vi "e.gate Cleanup.vi"(8 "error in (no error)":errorcluster, 11 "e.gate Configuration":T1 {"dActTimeToSecondFactor" format="%#.10f"; "StartTimeToDayFactor" format="%#.10f"; "BufferFillRate" format="%#_10f"}) -> (0 "error out":errorcluster)   [LabVIEW 2016]
doc: "<B>AMC - Analytik & Messtechnik GmbH Chemnitz</B>\n\nLabVIEW Drivers for e.gate / e.pac series from Gantner Instruments\n\nThis VI closes the TCP/IP interface specified by <B>connection ID</B>. An incoming error is ignored but forwarded."
uses:
  e.gate Configuration.ctl
  e.gate Channel Data.ctl
  e.gate Data Type.ctl
  e.gate Protocol Type.ctl
  e.gate Module  Data.ctl
  e.gateHSP_DLLhandle.ctl
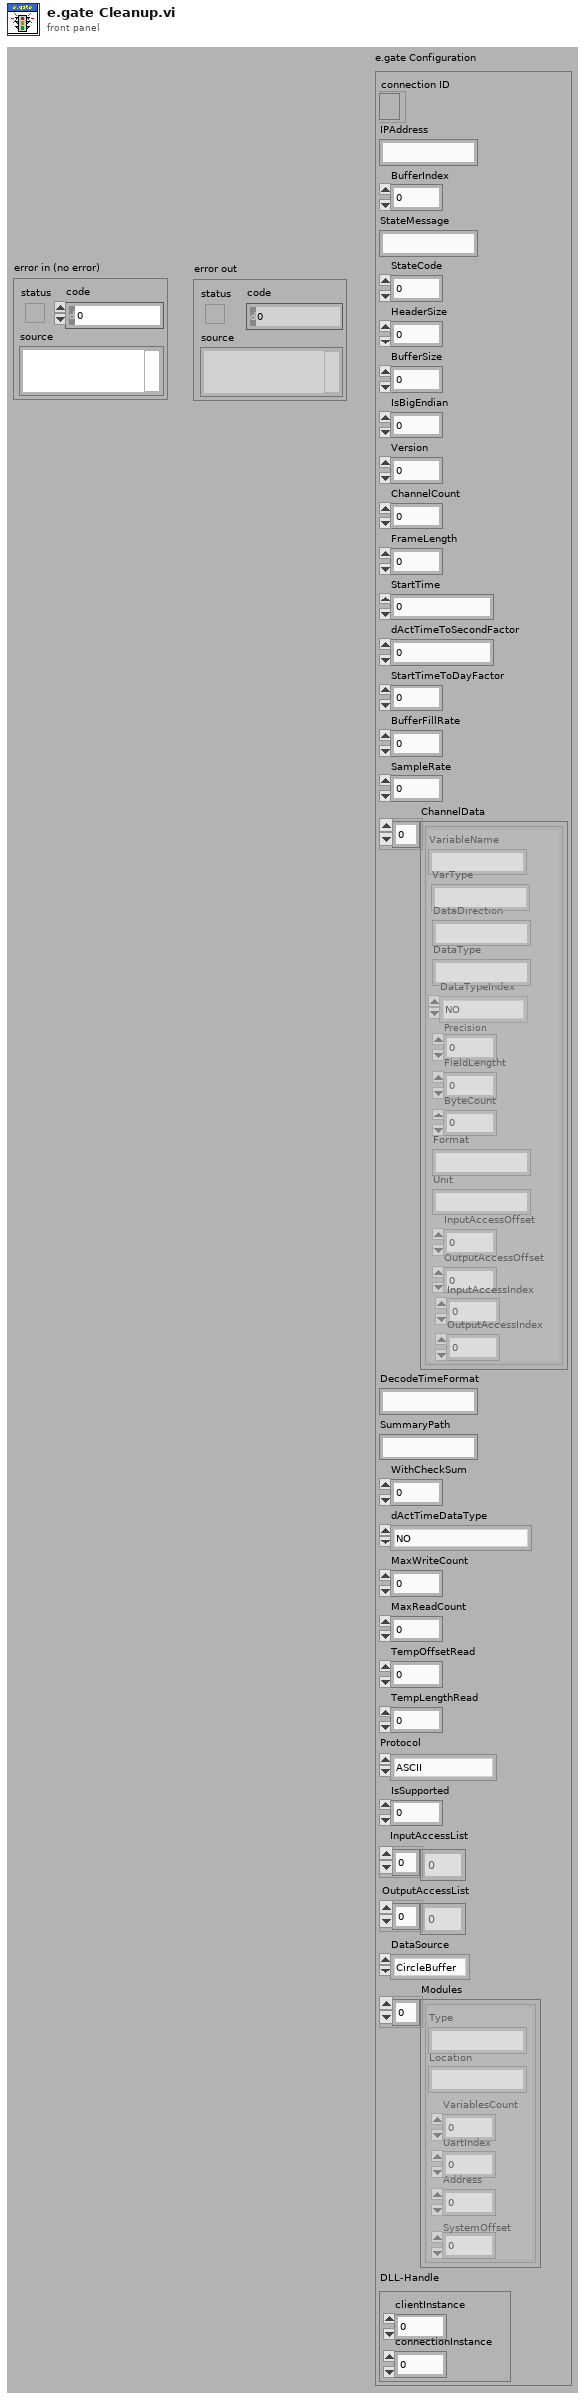
[diagram p1: front panel]
types:
  T1 = typedef "e.gate Configuration.ctl" = cluster{"connection ID":refnum<k5>, "IPAddress":string, "BufferIndex":i32, "StateMessage":string, "StateCode":i8, "HeaderSize":i32, "BufferSize":i32, "IsBigEndian":i32, "Version":i32, "ChannelCount":i32, "FrameLength":i32, "StartTime":dbl, "dActTimeToSecondFactor":dbl, "StartTimeToDayFactor":dbl, "BufferFillRate":dbl, "SampleRate":dbl, "ChannelData":T2[], "DecodeTimeFormat":string, "SummaryPath":string, "WithCheckSum":i32, "dActTimeDataType":T3, "MaxWriteCount":i32, "MaxReadCount":i32, "TempOffsetRead":i32, "TempLengthRead":i32, "Protocol":T4, "IsSupported":i32, "InputAccessList":i32[], "OutputAccessList":i32[], "DataSource":enum16{"CircleBuffer", "test.con Logger", "test.con Archive"}, "Modules":T5[], "DLL-Handle":T6}
  T2 = typedef "e.gate Channel Data.ctl" = cluster{"VariableName":string, "DataDirection":string, "DataType":string, "DataTypeIndex":T3, "Precision":i16, "FieldLengtht":i16, "ByteCount":i32, "Format":string, "Unit":string, "InputAccessOffset":i32, "OutputAccessOffset":i16, "InputAccessIndex":i16, "OutputAccessIndex":i16, "VarType":string}
  T3 = typedef "e.gate Data Type.ctl" = enum16{"NO", "BOOL", "SINT8", "USINT8", "SINT16", "USINT16", "SINT32", "USINT32", "FLOAT", "SET8", "SET16", "SET32", "DOUBLE", "SINT64", "USINT64", "SET64"}
  T4 = typedef "e.gate Protocol Type.ctl" = enum16{"ASCII", "HighspeedPort Online", "HighspeedPort Buffer", "eGateHighspeedPortDLL "}
  T5 = typedef "e.gate Module  Data.ctl" = cluster{"Type":string, "Location":string, "VariablesCount":i16, "UartIndex":i16, "Address":i16, "SystemOffset":i16}
  T6 = typedef "e.gateHSP_DLLhandle.ctl" = cluster{"clientInstance":i32, "connectionInstance":i32}
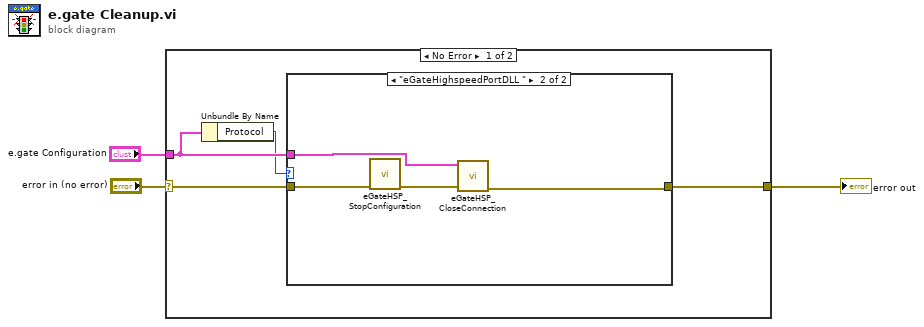
[diagram p0: block diagram]
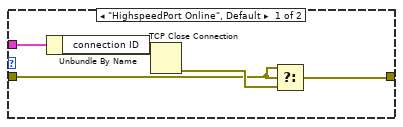
[diagram p2: hidden frame]
diagram:
  n1 = case shown="No Error" "error in (no error)" {
    selector: "error in (no error)" -> [w6 w17]
    tunnel: [w7 w17] -> w3
    tunnel: "e.gate Configuration" -> [w5 _]
    frame No Error {
      n2 = Unbundle By Name(w5) -> ("Protocol"=w4:T4)
      n3 = case shown="\"eGateHighspeedPortDLL \"" w4 {
        tunnel: [w12 w14] -> w7
        tunnel: w6 -> [w9 w16]
        tunnel: w5 -> [w8 w13]
        frame "HighspeedPort Online", Default {
          n4 = Unbundle By Name(w8) -> ("connection ID"=w11:refnum<k5>)
          n5 = TCP Close Connection(connection ID=w11) -> (error out=w10:errorcluster)  [unwired: 1 in, 2 out]
          n6 = Select(t=w9, s=w9, f=w10) -> (s? t:f=w12:errorcluster)
        }
        frame "eGateHighspeedPortDLL " {
          n7 = call "eGateHSP_StopConfiguration.vi"("Fehler (Eingang, kein Fehler)"=w16) -> ("Fehler (Ausgang)"=w15:errorcluster)  [unwired: 10 in]
          n8 = call "eGateHSP_CloseConnection.vi"("Fehler (Eingang, kein Fehler)"=w15, "e.gate Configuration"=w13) -> ("Fehler (Ausgang)"=w14:errorcluster)  [unwired: 9 in]
        }
      }
    }
    frame Error {
    }
  }
  "error out" <- w3
